vi "Node - Connect.vi"(8 "error in (no error)":errorcluster, 11 "Node Data In":T1) -> (0 "error out":errorcluster, 3 "Node Data Out":T1)   [LabVIEW 2016, in "PXImc Router.lvlib"]
uses:
  PXImc Router.lvlib
  Controls/Node Data.ctl
  <vilib>/NI Veristand/VeriStand Data/Byte Buffer/Byte Buffer.lvclass
  Controls/Node/Node - PXImc Parameters.ctl
  Controls/Node/Node - Writer Data.ctl
  Controls/Node/Node Ch Properties.ctl
  Controls/Data Type.ctl
  Controls/Node/Node - Readers Data.ctl
  Controls/Node/Node - Reader Data.ctl
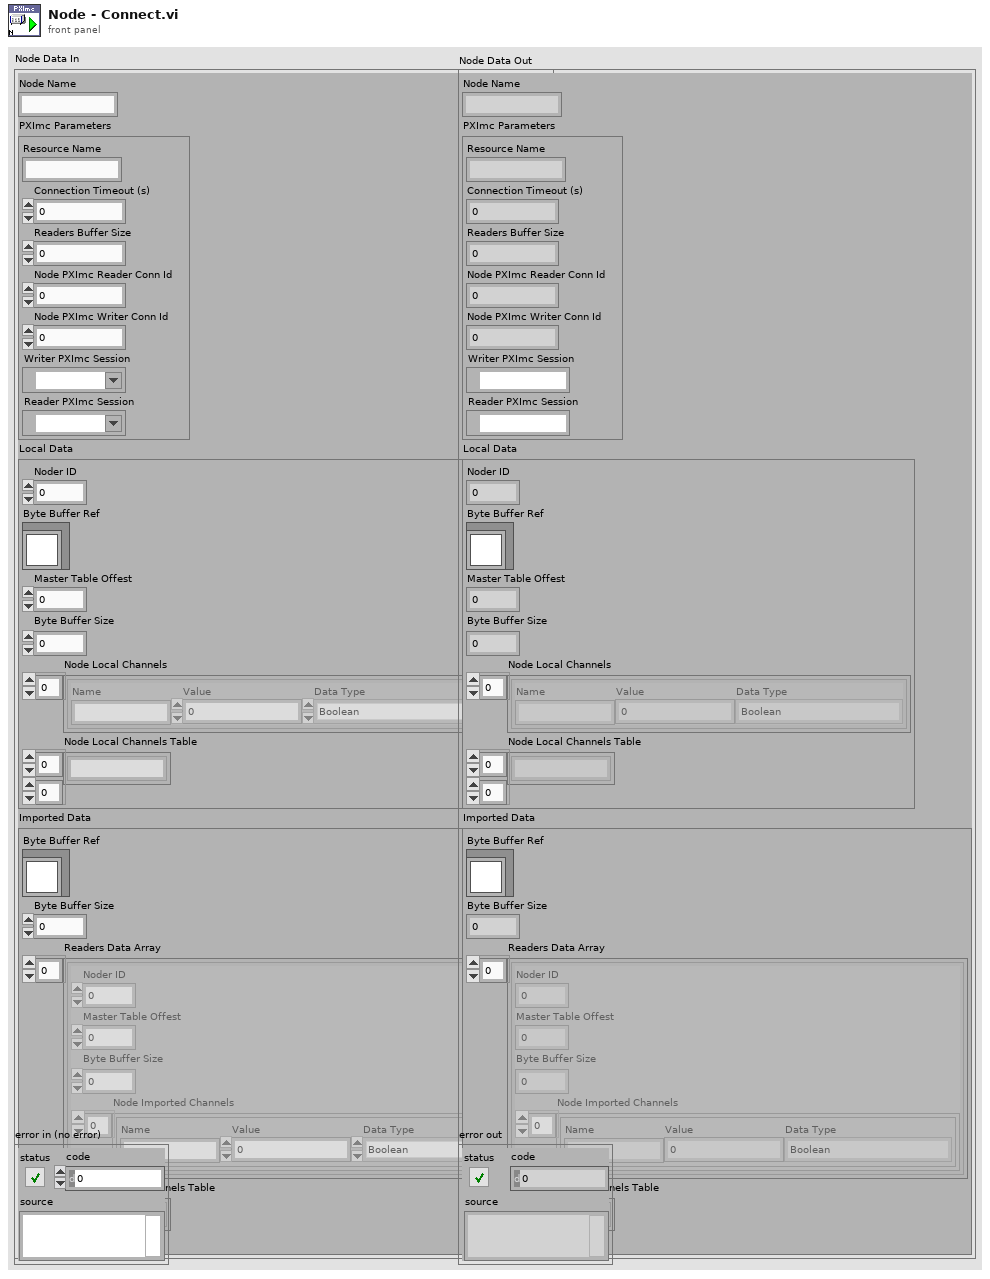
[diagram p1: front panel]
types:
  T1 = typedef "PXImc Router.lvlib/Node Data.ctl" = cluster{"Node Name":string, "PXImc Parameters":T2, "Local Data":T3, "Imported Data":T6}
  T2 = typedef "PXImc Router.lvlib/Node - PXImc Parameters.ctl" = cluster{"Resource Name":string, "Connection Timeout (s)":dbl, "Readers Buffer Size":u64, "Node PXImc Reader Conn Id":u16, "Node PXImc Writer Conn Id":u16, "Writer PXImc Session":refnum<k21>, "Reader PXImc Session":refnum<k21>}
  T3 = typedef "PXImc Router.lvlib/Node - Writer Data.ctl" = cluster{"Noder ID":u32, "Byte Buffer Ref":refnum<class "Byte Buffer.lvclass">, "Master Table Offest":u32, "Byte Buffer Size":u32, "Node Local Channels":T4[], "Node Local Channels Table":string[][]}
  T4 = typedef "PXImc Router.lvlib/Node Ch Properties.ctl" = cluster{"Name":string, "Value":dbl, "Data Type":T5}
  T5 = typedef "PXImc Router.lvlib/Data Type.ctl" = enum16{"Boolean", "SGL", "DBL", "I8", "I16", "I32", "I64", "U8", "U16", "U32", "U64"}
  T6 = typedef "PXImc Router.lvlib/Node - Readers Data.ctl" = cluster{"Byte Buffer Ref":refnum<class "Byte Buffer.lvclass">, "Byte Buffer Size":u64, "Readers Data Array":T7[], "Node Imported Channels Table":string[][]}
  T7 = typedef "PXImc Router.lvlib/Node - Reader Data.ctl" = cluster{"Noder ID":u32, "Master Table Offest":u32, "Byte Buffer Size":u64, "Node Imported Channels":T4[]}
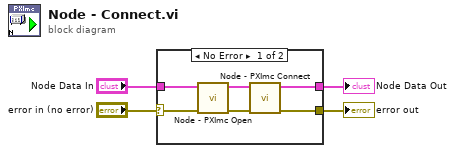
[diagram p0: block diagram]
diagram:
  n1 = case shown="No Error" "error in (no error)" {
    selector: "error in (no error)" -> [w5 w11]
    tunnel: [w10 w12] -> w4
    tunnel: [w9 w11] -> w3
    tunnel: "Node Data In" -> [w8 w12]
    frame No Error {
      n2 = call "Node - PXImc Open.vi"("error in (no error)"=w5, "Node Data In in"=w8) -> ("error out"=w6:errorcluster, "Node Data In out"=w7:T1)  [unwired: 8 in]
      n3 = call "Node - PXImc Connect.vi"("error in (no error)"=w6, "Node Data In in"=w7) -> ("error out"=w9:errorcluster, "Node Data In out"=w10:T1)  [unwired: 8 in]
    }
    frame Error {
    }
  }
  "Node Data Out" <- w4
  "error out" <- w3
